vi "Timer_StopInternal.vi"(11 "in Timer":T1 {"Accumulated TIme" format="%13.5p"; "StartTime" format="%13.5p"}) -> (3 "out Timer":T1 {"Accumulated TIme" format="%13.5p"; "StartTime" format="%13.5p"})   [LabVIEW 2019, in "Trajectory_Library.lvlib"]
doc: "THIS IS AN INTERNAL ROUTINE. DO NOT USE.\n \nStop the timer. This computes the time as of now and clears the running flag, causing all subsequent time requests to be read from the accumulated time rather than looking at the system clock.\n\nInputs:\n - Timer -- The Timer data cluster\n\nOutputs:\n - Timer -- The modified Timer data cluster"
uses:
  Trajectory_Library.lvlib
  TIMER.ctl
  Util_GetTime.vi
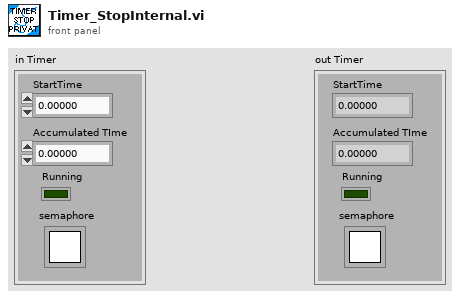
[diagram p1: front panel]
types:
  T1 = typedef "Trajectory_Library.lvlib/TIMER.ctl" = cluster{"StartTime":dbl, "Accumulated TIme":dbl, "Running":bool, "semaphore":T2}
  T2 = typedef "Semaphore RefNum" = refnum<k1>
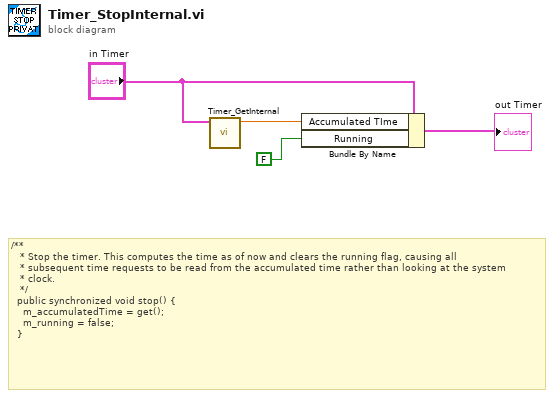
[diagram p0: block diagram]
diagram:
  # "/**\n   * Stop the timer. This computes the time as of now and clears the running flag, causing all\n   * subsequent time requests to be read from the accumulated time rather than looking at the system\n   * clock.\n   */\n  public synchronized void stop() {\n    m_accumulatedTime = get();\n    m_running = false;\n  }"
  n1 = call "Timer_GetInternal.vi"("TIMER"="in Timer") -> ("CurrentTImer"=w2:dbl)  [unwired: 9 in, 1 out]
  n2 = Bundle By Name(cluster="in Timer", "Accumulated TIme"=w2, "Running"=FALSE) -> (→"out Timer":T1)
